vi "Pre_Build.vi"(8 "error in (no error)":errorcluster, 11 "Build in":refnum<class "AB_Build.lvclass">) -> (0 "error out":errorcluster, 3 "Build out":refnum<class "AB_Build.lvclass">)   [LabVIEW 2020, in "AB_Deployment.lvlib"]
uses:
  <vilib>/AppBuilder/AB_Classes/Deployment/AB_Deployment.lvlib
  <vilib>/AppBuilder/AB_Classes/Build/AB_Build.lvclass
  <vilib>/AppBuilder/AB_Classes/Destination/AB_Destination.lvclass
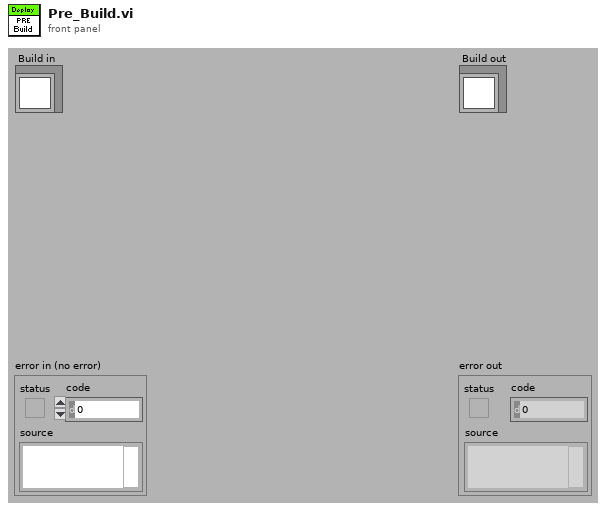
[diagram p1: front panel]
types:
  T1 = typedef "AB_Build.ctl" = cluster{"buildSpecName":string, "buildSpecDescription":string, "destinations":refnum<class "AB_Destination.lvclass">[], "exclusionOption":T2, "defaultLanguage":string, "supportedLanguages":string[], "excludedDirectories":path[], "buildContext":refnum<vi>, "buildObject":T3, "preview":bool, "programatic":bool, "progressBarEvents":T4, "userLog_Path":path, "preActionID":string, "preAction_Path":path, "postActionID":string, "postAction_Path":path, "eng_checkForBrokenVIs?":bool, "eng_verboseLinkerErrors?":bool, "localDest_Path":path, "targetDest_Path":path, "removeVIObject":u16, "cache":refnum<class "PreviewCache.lvclass">, "use cache":bool, "previewCache_ID":string, "buildCache_ID":string, "eng_TempLocalDest_Path":path, "eng_collectDependencies?":bool, "versionInfo":cluster{"buildVersion":cluster{"major":u16, "minor":u16, "patch":u16, "build":u16}, "autoIncrement":bool}, "eng_enableVIChecksums":bool}
  T2 = typedef "AB_Exclusion_Option.ctl" = cluster{"typedefs":bool, "polymorphicVIs":bool, "unusedLibraryItems":bool, "modifyLibraryFile":bool, "edit-timeDependencies":bool, "inlineVIs":bool, "dependent PPLs":bool, "dependent DLLs":bool}
  T3 = typedef "ItemRef.ctl" = u64
  T4 = typedef "provcom_ProgressBar_Events.ctl" = cluster{"newJob":refnum<user-event>, "newItem":refnum<user-event>, "errorMsg":T5, "cancel":refnum<user-event>}
  T5 = typedef "mxLvBuildError.ctl" = refnum<user-event>
  T6 = typedef "AB_Destination.ctl" = cluster{"destName":string, "path":path, "libraryName":string, "preserveHierarchy":bool, "eng_inBuild":bool, "eng_libraryReference":refnum<vi>, "eng_restictAddToNewLibrary":bool}
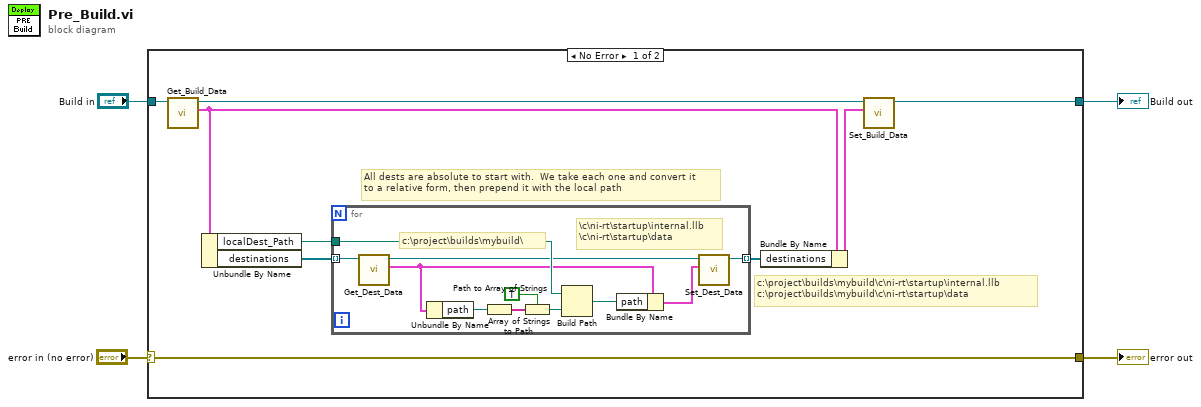
[diagram p0: block diagram]
diagram:
  n1 = case shown="No Error" "error in (no error)" {
    selector: "error in (no error)" -> [w13 w25]
    tunnel: [w5 w26] -> w4
    tunnel: "Build in" -> [w9 w26]
    tunnel: [w13 w25] -> w2
    frame No Error {
      # "c:\\project\\builds\\mybuild\\c\\ni-rt\\startup\\internal.llb\nc:\\project\\builds\\mybuild\\c\\ni-rt\\startup\\data"
      # "All dests are absolute to start with.  We take each one and convert it\nto a relative form, then prepend it with the local path"
      n2 = call <vilib>:"Get_Build_Data.vi"("Class in"=w9) -> ("data"=w11:T1, "Class out"=w10:refnum<class "AB_Build.lvclass">)  [unwired: 1 in, 8 out]
      n3 = Unbundle By Name(w11) -> ("localDest_Path"=w8:path, "destinations"=w12:refnum<class "AB_Destination.lvclass">[])
      n4 = for {
        tunnel: w12 -> [w18] mode=indexing
        tunnel: w8 -> [w21]
        tunnel: [w14] -> w6 mode=indexing
        # "\\c\\ni-rt\\startup\\internal.llb\n\\c\\ni-rt\\startup\\data"
        # "c:\\project\\builds\\mybuild\\"
        n5 = call <vilib>:"Get_Dest_Data.vi"("Class in"=w18) -> ("destName"=w17:T6, "Class out"=w16:refnum<class "AB_Destination.lvclass">)  [unwired: 1 in, 8 out]
        n6 = Unbundle By Name(w17) -> ("path"=w24:path)
        n7 = Path to Array of Strings(0:w24) -> (2:w23:string[])  [unwired: 1 out]
        n8 = Array of Strings to Path(0:w23, 1:TRUE ("relative")) -> (2:w20:path)
        n9 = Build Path(base path=w21, name or relative path=w20) -> (appended path=w19:path)
        n10 = Bundle By Name(cluster=w17, "path"=w19) -> (w15:T6)
        n11 = call <vilib>:"Set_Dest_Data.vi"("destName"=w15, "Class in"=w16) -> ("Class out"=w14:refnum<class "AB_Destination.lvclass">)  [unwired: 1 in, 8 out]
      }
      n12 = Bundle By Name(cluster=w11, "destinations"=w6) -> (w7:T1)
      n13 = call <vilib>:"Set_Build_Data.vi"("data"=w7, "Class in"=w10) -> ("Class out"=w5:refnum<class "AB_Build.lvclass">)  [unwired: 1 in, 8 out]
    }
    frame Error {
    }
  }
  "error out" <- w2
  "Build out" <- w4
